vi "EstPostureFromWheelSpd.vi"(0 "differential steering frame in":refnum<class "NI_Robotics_Differential Steering Frame.lvclass">, 1 "reinit?":bool, 5 "Wheel Velocity":T4, 7 "Robot Configuration":T1={"wheel parameters"={"wheel radius"=0.05, "gear ratio"=1.0, "forward rotation direction"=0}, "wheel separation"=0.19, "Encoder Pulse Per Rev"=1856.0, "Update Period (sec)"=0.02, "Initial posture frame"=[0.0, 0.0, 0.0]} {"wheel parameters"."forward rotation direction" items=["Clockwise", "Counterclockwise"]}, 11 "error in (no error)":errorcluster) -> (4 "steering frame out":refnum<class "NI_Robotics_Steering Frame.lvclass">, 6 "estimated steering frame posture":dbl[](array[numeric]), 15 "error out":errorcluster)   [LabVIEW 2016]
uses:
  <vilib>/robotics/Steering/Steering Frame/NI_Robotics_Steering Frame.lvclass
  <vilib>/robotics/Steering/Differential Steering Frame/NI_Robotics_Differential Steering Frame.lvclass
  C:/Program Files (x86)/National Instruments/LabVIEW 2016/vi.lib/robotics/Steering/Steering Frame/NI_Robotics_Steering Frame.lvclass
  MotorControl/Configurations.ctl
  <vilib>/robotics/Steering/Wheel/Wheel Parameters.ctl
  <vilib>/robotics/Steering/Wheel/Rotation Direction.ctl
  <vilib>/robotics/Steering/Steering Frame/Get Steering Frame Velocity from Motors.vi
  C:/Program Files (x86)/National Instruments/LabVIEW 2016/vi.lib/robotics/Steering/Special Steering Frame/NI_Robotics_Special Steering Frame.lvclass
  <vilib>/robotics/Steering/Wheel/NI_Robotics_Wheel.lvclass
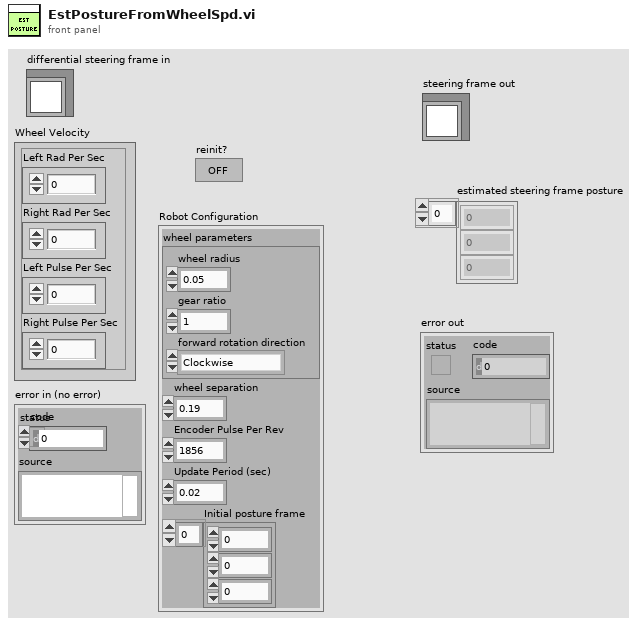
[diagram p1: front panel]
types:
  T1 = typedef "Configurations.ctl" = cluster{"wheel parameters":T2, "wheel separation":dbl, "Encoder Pulse Per Rev":dbl, "Update Period (sec)":dbl, "Initial posture frame":dbl[]}
  T2 = typedef "NI_Robotics_Wheel.lvclass/Wheel Parameters.ctl" = cluster{"wheel radius":dbl, "gear ratio":dbl, "forward rotation direction":T3}
  T3 = typedef "NI_Robotics_Wheel.lvclass/Rotation Direction.ctl" = u16
  T4 = cluster{"Left Rad Per Sec":dbl, "Right Rad Per Sec":dbl, "Left Pulse Per Sec":dbl, "Right Pulse Per Sec":dbl}
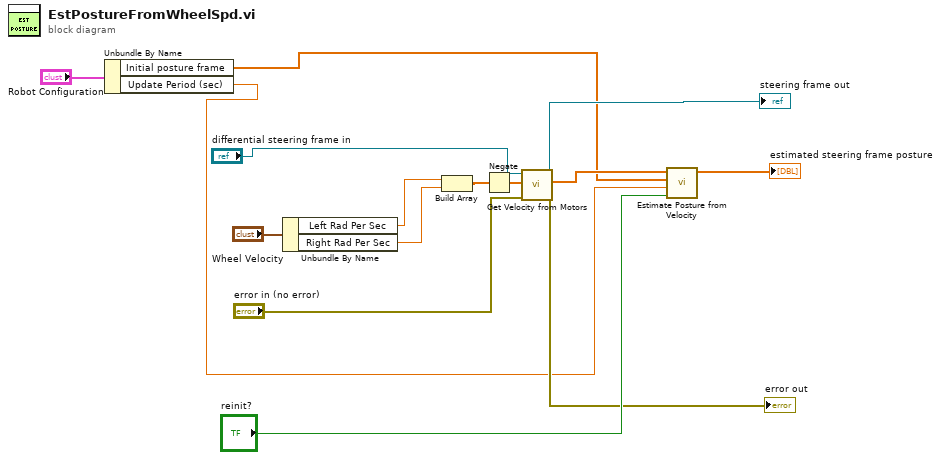
[diagram p0: block diagram]
diagram:
  n1 = Unbundle By Name("Robot Configuration") -> ("Initial posture frame"=w2:dbl[], "Update Period (sec)"=w1:dbl)
  n2 = Unbundle By Name("Wheel Velocity") -> ("Left Rad Per Sec"=w11:dbl, "Right Rad Per Sec"=w10:dbl)
  n3 = Build Array(w11, w10) -> (w14:dbl[])
  n4 = Negate(x=w14) -> (-x=w15:dbl[])
  n5 = call-poly <vilib>:"Get Velocity from Motors.vi"("error in (no error)"="error in (no error)", "ccw motor velocity states"=w15, "steering frame in"="differential steering frame in") -> ("error out"=→"error out":errorcluster, "estimated steering frame velocity"=w13:dbl[], "steering frame out"=→"steering frame out":refnum<class "NI_Robotics_Differential Steering Frame.lvclass">)  [unwired: 6 in]
  n6 = call "Estimate Posture from Velocity.vi"("initialize"="reinit?", "dt (s)"=w1, "initial posture"=w2, "estimated steering frame velocity"=w13) -> ("estimated steering frame posture"=→"estimated steering frame posture":dbl[])  [unwired: 7 in]
